vi "Run.vi"(8 "error in (no error)":errorcluster, 11 "Application in":refnum<class "Application.lvclass">) -> (0 "error out":errorcluster, 3 "Application out":refnum<class "Application.lvclass">)   [LabVIEW 2010, in "Application.lvclass"]
doc: "This VI contains the main architecture for all Applications. It uses the channeling pattern to ensure that each implementation will follow the same basic steps: Setup, Execute, Shutdown, Handle Error."
uses:
  Application.lvclass
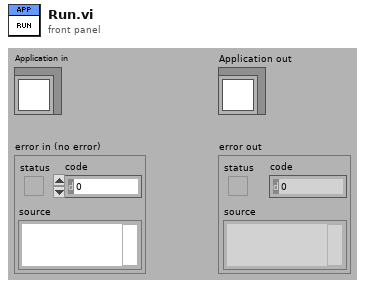
[diagram p1: front panel]
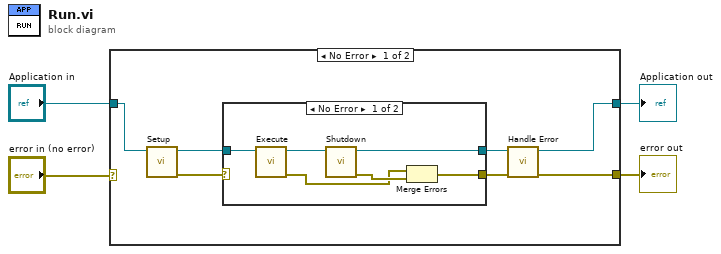
[diagram p0: block diagram]
diagram:
  n1 = case shown="No Error" "error in (no error)" {
    selector: "error in (no error)" -> [_ w21]
    tunnel: [w6 w21] -> w3
    tunnel: [w5 w20] -> w1
    tunnel: "Application in" -> [w10 w20]
    frame No Error {
      n2 = call-dynamic "Setup.vi"("Application in"=w10) -> ("error out"=w11:errorcluster, "Application out"=w9:refnum<class "Application.lvclass">)  [unwired: 9 in]
      n3 = case shown="No Error" w11 {
        selector: w11 -> [_ w19]
        tunnel: w9 -> [w17 w18]
        tunnel: [w14 w19] -> w7
        tunnel: [w13 w18] -> w8
        frame No Error {
          n4 = call-dynamic "Execute.vi"("Application in"=w17) -> ("error out"=w12:errorcluster, "Application out"=w16:refnum<class "Application.lvclass">)  [unwired: 9 in]
          n5 = call-dynamic "Shutdown.vi"("Application in"=w16) -> ("error out"=w15:errorcluster, "Application out"=w13:refnum<class "Application.lvclass">)  [unwired: 9 in]
          n6 = Merge Errors "Merge Errors"(w12, w15) -> (w14:errorcluster)
        }
        frame Error {
        }
      }
      n7 = call-dynamic "Handle Error.vi"("error in (no error)"=w7, "Application in"=w8) -> ("error out"=w6:errorcluster, "Application out"=w5:refnum<class "Application.lvclass">)  [unwired: 8 in]
    }
    frame Error {
    }
  }
  "error out" <- w3
  "Application out" <- w1
